vi "Wait for mode change.vi"(7 "error constant":errorcluster, 9 "Timeout (ms)":i32=-1, 10 "Mode":refnum<user-event>) -> (0 "error constant 2":errorcluster)   [LabVIEW 2023, in "Application.lvlib"]
uses:
  Application.lvlib
  Mode.ctl
panel:
  out "Event Started?":bool
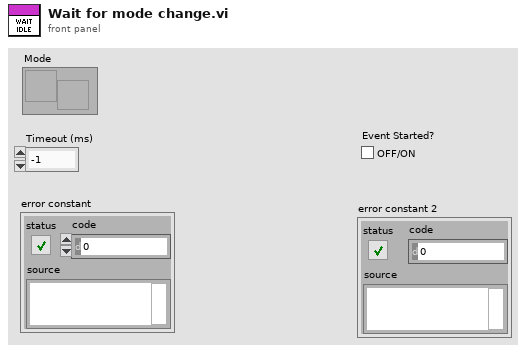
[diagram p1: front panel]
types:
  T1 = typedef "Application.lvlib/Mode.ctl" = enum16{"Idle", "Cancel", "Live", "Stream", "Autofocus", "Z-Stack"}
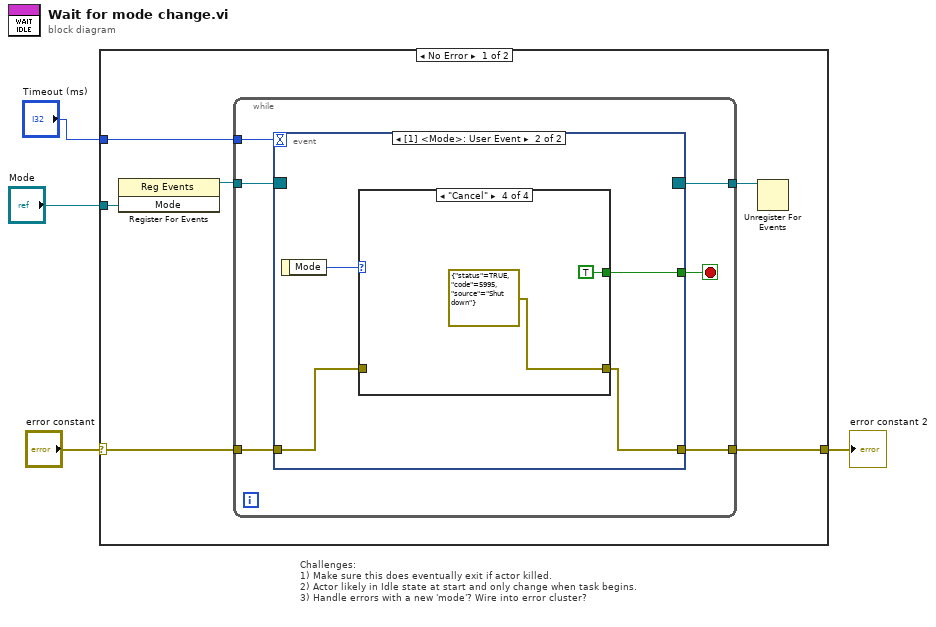
[diagram p0: block diagram]
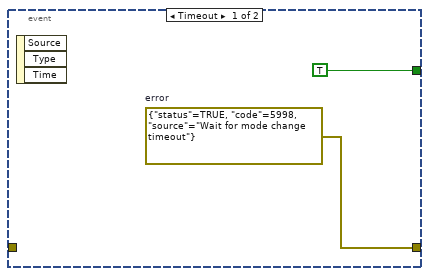
[diagram p2: hidden frame]
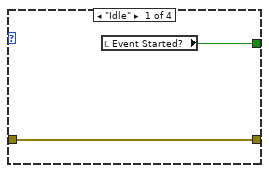
[diagram p3: hidden frame]
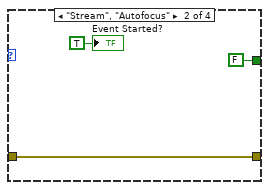
[diagram p4: hidden frame]
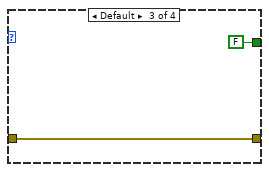
[diagram p5: hidden frame]
diagram:
  # "Challenges:\n1) Make sure this does eventually exit if actor killed.\n2) Actor likely in Idle state at start and only change when task begins.\n3) Handle errors with a new 'mode'? Wire into error cluster?"
  n1 = case shown="No Error" "error constant" {
    selector: "error constant" -> [w9 w32]
    tunnel: "Timeout (ms)" -> [w10 _]
    tunnel: [w8 w32] -> w2
    tunnel: "Mode" -> [w6 _]
    frame No Error {
      n2 = register-events(w6) -> (reference out=w5:refnum<event-registration>)  [unwired: 2 in, 1 out]
      n3 = while {
        tunnel: w5 -> [w16]
        tunnel: w10 -> [w14]
        tunnel: w9 -> [w13]
        tunnel: [w12] -> w8
        tunnel: [w11] -> w7
        stop <- w15 stop-if-true
        n4 = event shown="[1] <Mode>: User Event" {
          selector: w16 -> [_ _]
          dyn-events: [_ _] -> w11
          timeout: w14 -> [_ _]
          tunnel: [TRUE ("Event Started?") w21] -> w15
          tunnel: w13 -> [_ w20]
          tunnel: [w17 w19] -> w12
          event Timeout {
            w17 = errorcluster {"status"=TRUE, "code"=5998, "source"="Wait for mode change timeout"}  # error
            n5 = event-data() -> ()  [unwired: 1 in, 3 out]
          }
          event User Event {
            n6 = event-data() -> ("Mode"=w22:T1)  [unwired: 1 in]
            n7 = case shown="\"Cancel\"" w22 {
              tunnel: [w24 FALSE ("Event Started?") FALSE ("Event Started?") TRUE ("Event Started?")] -> w21
              tunnel: w20 -> [w23 w25 w28 _]
              tunnel: [w23 w25 w28 errorcluster {"status"=TRUE, "code"=5995, "source"="Shut down"} ("error constant")] -> w19
              frame "Idle" {
                n8 = local read "Event Started?"() -> (w24:bool)
              }
              frame "Stream", "Autofocus" {
                "Event Started?" <- TRUE ("Event Started?")
              }
              frame Default {
              }
              frame "Cancel" {
              }
            }
          }
        }
      }
      n9 = Unregister For Events(event registration refnum=w7) -> ()  [unwired: 1 in, 1 out]
    }
    frame Error {
    }
  }
  "error constant 2" <- w2
